vi "Splash Screen.vi"(9 "error in (no error)":errorcluster) -> (1 "error out":errorcluster)   [LabVIEW 2009]
uses:
  <vilib>/Utility/cursorutil.llb/Set Cursor (Icon Pict).vi
panel:
  out "Click to Continue...":bool
  out "SW Ver":string caption="Version:"
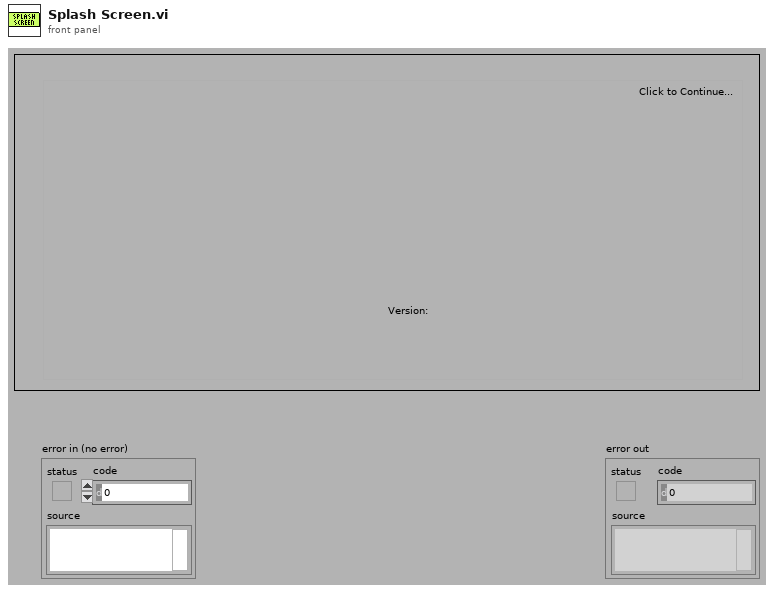
[diagram p1: front panel]
types:
  T1 = enum32{"invalid app kind", "Development System", "Run Time System", "Student Edition", "Embedded LabVIEW", "Evaluation", "Custom"}
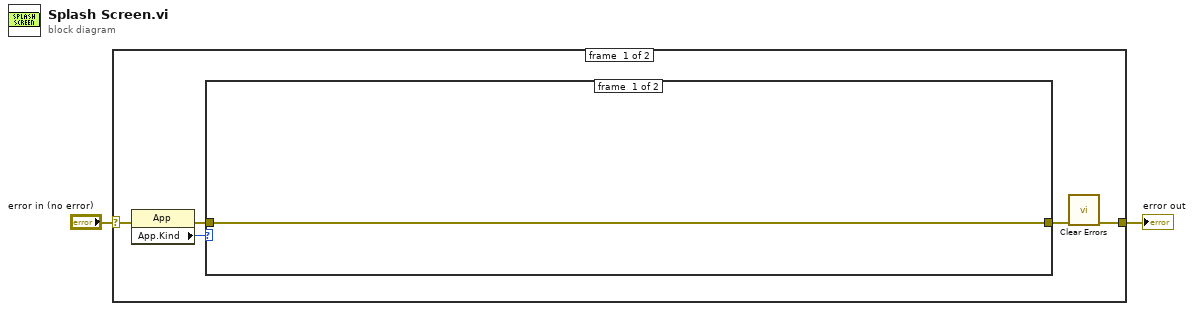
[diagram p0: block diagram]
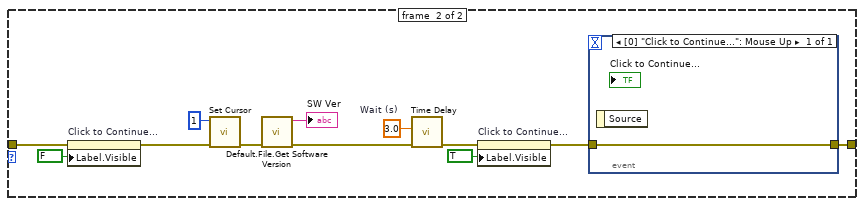
[diagram p2: hidden frame]
diagram:
  n1 = case shown="No Error" "error in (no error)" {
    selector: "error in (no error)" -> [w7 w22]
    tunnel: [w3 w22] -> w1
    frame #0 {
      n2 = property class="App"(error in=w7) -> (error out=w6:errorcluster, "App.Kind"=w5:T1)  [unwired: 1 in, 1 out]
      n3 = case shown="\"Run Time System\"" w5 {
        tunnel: [w8 w13] -> w4
        tunnel: w6 -> [w8 w9]
        frame #0 {
        }
        frame #1 {
          w19 = 3.0  # Wait (s)
          n4 = property on="Click to Continue..." class="Bool (strict)"(error in=w9, "Label.Visible"=FALSE) -> (error out=w18:errorcluster)  [unwired: 1 in, 1 out]
          n5 = call-poly <vilib>:"Set Cursor.vi"("error in (no error)"=w18, "icon"=u16 1) -> ("error out"=w12:errorcluster)  [unwired: 1 in, 8 out]
          n6 = call <userlib>:"Default.File.Get Software Version.vi"("error in (no error)"=w12) -> ("error out"=w11:errorcluster, "Softare Version:"=→"SW Ver":string)  [unwired: 9 out]
          n7 = call "Time Delay"("error in (no error)"=w11, "Delay Time (s)"=w19) -> ("error out"=w15:errorcluster)  [unwired: 1 in, 8 out]
          n8 = property on="Click to Continue..." class="Bool (strict)"(error in=w15, "Label.Visible"=TRUE) -> (error out=w14:errorcluster)  [unwired: 1 in, 1 out]
          n9 = event shown="[0] \"Click to Continue...\": Mouse Up" {
            selector: _ -> [_]
            dyn-events: _ -> [_]
            timeout: _ -> [_]
            tunnel: w14 -> [w21]
            tunnel: [w21] -> w13
            event [0] "Click to Continue...": Mouse Up {
              n10 = event-data() -> ()  [unwired: 2 out]
            }
          }
        }
      }
      n11 = call <vilib>:"Clear Errors.vi"("error in (no error)"=w4) -> ("error out"=w3:errorcluster)  [unwired: 6 in]
    }
    frame #1 {
    }
  }
  "error out" <- w1
